vi "DriveSetGyroZero.vi"(8 "error in (no error)":errorcluster, 11 "GyroZero":dbl) -> (0 "error out":errorcluster)   [LabVIEW 2020]
doc: "Set GyroZero\n\nInputs:\n--GyroZero--Double--set gyro zero"
uses:
  DriveGlobal.vi
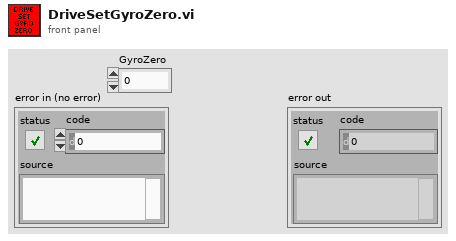
[diagram p1: front panel]
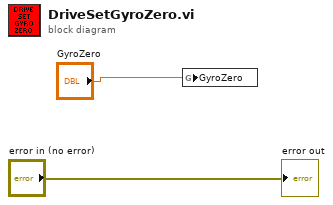
[diagram p0: block diagram]
diagram:
  n1 = global write "DriveGlobal.vi" "GyroZero"("GyroZero") -> ()
  "error out" <- "error in (no error)"
